vi "Set Path Values.vi"(7 "Target (Process)":T1 items=["Process", "User", "Machine"], 8 "Error In":errorcluster, 11 "Values[]":string[](array[string])) -> (0 "Error Out":errorcluster)   [LabVIEW 2023, in "SLL Environment Variable.lvlib"]
doc: "Set the <B>Values[]</B> to <B>Path</B> variable in the target environment."
uses:
  SLL Environment Variable.lvlib
  _Typedef/Target Environment Enum.ctl
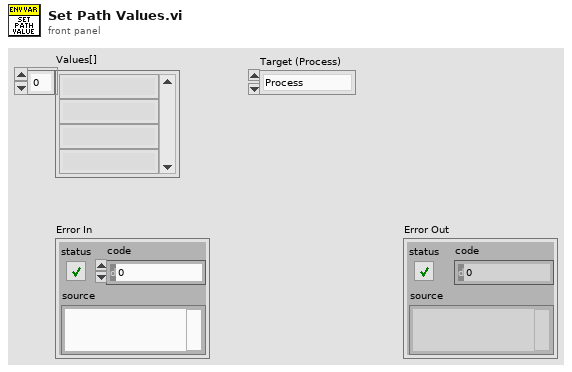
[diagram p1: front panel]
types:
  T1 = typedef "SLL Environment Variable.lvlib/Target Environment Enum.ctl" = i32
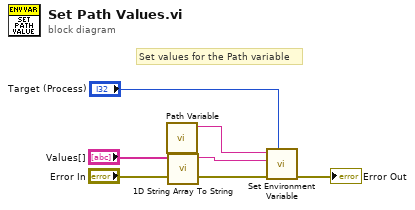
[diagram p0: block diagram]
diagram:
  # "Set values for the Path variable"
  n1 = call "Path Variable.vi"() -> ("Path Variable"=w1:string)  [unwired: 11 in]
  n2 = call "1D String Array To String.vi"("Array[]"="Values[]") -> ("String"=w6:string)  [unwired: 10 in]
  n3 = call "Set Environment Variable.vi"("Target (Process)"="Target (Process)", "Error In"="Error In", "Value"=w6, "Name"=w1) -> ("Error Out"=→"Error Out":errorcluster)  [unwired: 7 in]
